vi "Main.vi"() -> ()   [LabVIEW 2017]
doc: "The myRIO Project template acquires acceleration data from the onboard accelerometer and displays the changes of acceleration values in a waveform chart."
uses:
  ServoEnumControl.ctl
  ServoAbsAngleControl.ctl
  <vilib>/myRIO/Common/Instrument Driver Framework/myRIO v1.0/UART/vis/myRIO v1.0 Close UART.vi
  <vilib>/myRIO/Common/Instrument Driver Framework/Utilities/vis/FPGA Ref Manager.vi
  <vilib>/myRIO/Common/Instrument Driver Framework/myRIO v1.0/myRIO v1.0 Reset FPGA.vi
  <vilib>/myRIO/Common/Instrument Driver Framework/myRIO v1.0/IRQ/vis/myRIO v1.0 IRQ Info FGV.vi
  <vilib>/myRIO/Common/Instrument Driver Framework/myRIO v1.0/IRQ/vis/myRIO v1.0 Timer IRQ Info FGV.vi
  <vilib>/myRIO/Common/Instrument Driver Framework/myRIO v1.0/IRQ/vis/myRIO v1.0 ISR Agent.vi
  <vilib>/myRIO/Instrument Drivers/Utilities/Utilities.lvlib
panel:
  in  "Turn to":T1=-90 items=["-90°"=-90, "0°"=0, "+90°"=90]
  in  "Servo":T2
  out "Error":errorcluster
  in  "Stop":bool
  # "Test App: Turn and Grip Servos"
  # "Test four VI's\n\nServoInit.vi\nServoTurn.vi\nGripInit.vi\nGripDoIt.vi"
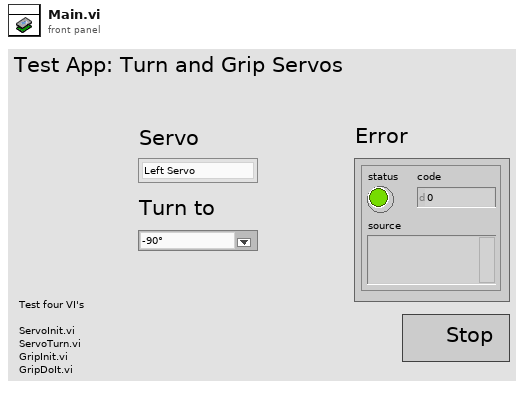
[diagram p1: front panel]
types:
  T1 = typedef "ServoAbsAngleControl.ctl" = i16
  T2 = typedef "ServoEnumControl.ctl" = enum16{"Left Servo", "Front Servo", "Right Servo"}
  T3 = typedef "PWM.lvlib/PWM Reference.ctl" = cluster{"myRIO Reference":T4, "PWM Channels Enum":T8, "PWM Configuration":T9}
  T4 = typedef "myRIO Generic Hardware Reference.ctl" = cluster{"myRIO Model":T5, "myRIO Hardware Reference":T6}
  T5 = typedef "Hardware Version Enum.ctl" = enum16{"Unknown", "myRIO-1900", "myRIO-1950", "roboRIO", "NI ELVIS RIO CM"}
  T6 = typedef "myRIO v1.0 Reference.ctl" = cluster{"Generic FPGA Reference":T7, "Allow multiple opens":bool}
  T7 = typedef "Generic FPGA Reference.ctl" = refnum<k20>
  T8 = typedef "PWM Channels Enum.ctl" = enum16{"Not Connected", "C/PWM0", "C/PWM1", "A/PWM0", "A/PWM1", "A/PWM2", "B/PWM0", "B/PWM1", "B/PWM2", "PWM/PWM0", "PWM/PWM1", "PWM/PWM2", "PWM/PWM3", "PWM/PWM4", "PWM/PWM5", "PWM/PWM6", "PWM/PWM7", "PWM/PWM8", "PWM/PWM9"}
  T9 = typedef "PWM.lvlib/PWM Configuration.ctl" = cluster{"Frequency":dbl, "Duty Cycle":dbl}
  T10 = cluster{T3[], "PWM Frequency":dbl, "b":dbl, "a":dbl}
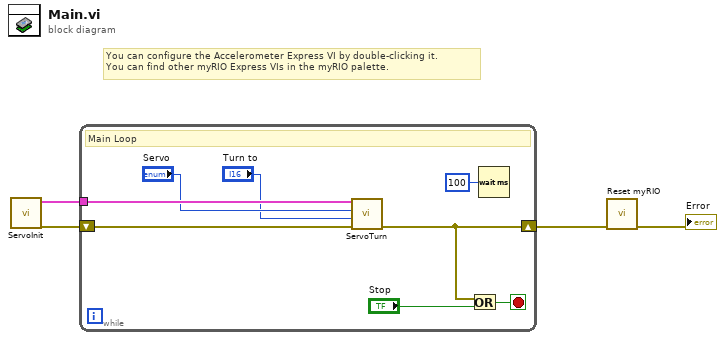
[diagram p0: block diagram]
diagram:
  # "You can configure the Accelerometer Express VI by double-clicking it.\nYou can find other myRIO Express VIs in the myRIO palette."
  n1 = call "ServoInit.vi"() -> ("error"=w2:errorcluster, "PWM channel cluster"=w1:T10)  [unwired: 6 in]
  n2 = while {
    shift-right: [w8] -> w4
    shift-left: w2 -> [w9]
    tunnel: w1 -> [w7]
    stop <- w11 stop-if-true
    # "Main Loop"
    n3 = call "ServoTurn.vi"("error in"=w9, "Turn to"="Turn to", "Servo Enum"="Servo", "PWM channel\n cluster"=w7) -> ("error out"=w8:errorcluster)  [unwired: 2 in, 1 out]
    n4 = Or(x=w8, y="Stop") -> (x .or. y?=w11:bool)
    n5 = Wait (ms)(milliseconds to wait=u32 100) -> ()  [unwired: 1 out]
  }
  n6 = call <vilib>:"Reset myRIO.vi"("error in (no error)"=w4) -> ("error out"=→"Error":errorcluster)  [unwired: 10 in]
